vi "Find Table Boundaries.vi"(8 "error in (no error)":errorcluster, 11 "Configuration in":refnum<class "Configuration.lvclass">) -> (0 "error out":errorcluster, 3 "Configuration out":refnum<class "Configuration.lvclass">)   [LabVIEW 2023, in "Configuration.lvlib" / "Configuration.lvclass"]
doc: "Search the raw signal list data for the device handle, read the row and column definition fields, this defines the boundary of the device defintion table."
uses:
  Library/Configuration.lvclass
  Library/Configuration.lvclass/Configuration.ctl
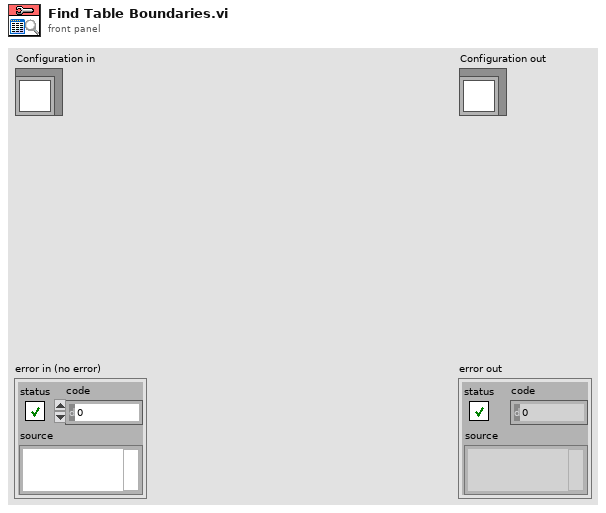
[diagram p1: front panel]
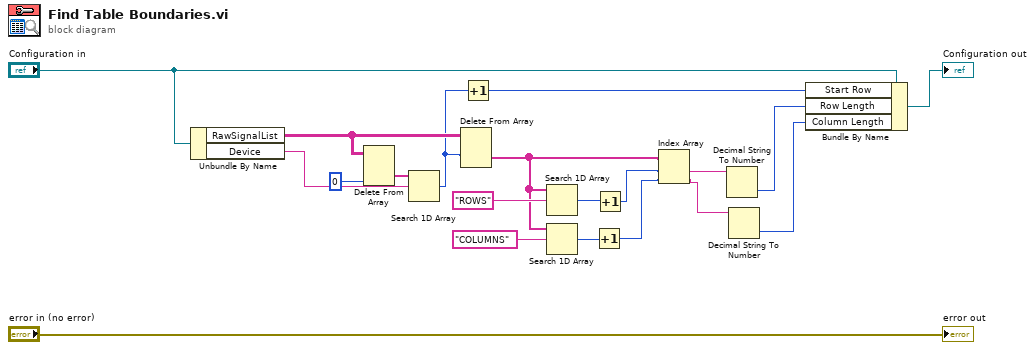
[diagram p0: block diagram]
diagram:
  n1 = Unbundle By Name("Configuration in") -> ("RawSignalList"=w17:string[][], "Device"=w1:string)
  n2 = Delete From Array(array=w17, index (col)=0 ("disabled index (col)")) -> (deleted portion=w18:string[])  [unwired: 2 in, 1 out]
  n3 = Search 1D Array(1D array=w18, element=w1) -> (index of element=w8:i32)  [unwired: 1 in]
  n4 = Delete From Array(array=w17, index (row)=w8) -> (deleted portion=w12:string[])  [unwired: 2 in, 1 out]
  n5 = Increment(x=w8) -> (x+1=w7:i32)
  n6 = Search 1D Array(1D array=w12, element="ROWS") -> (index of element=w14:i32)  [unwired: 1 in]
  n7 = Search 1D Array(1D array=w12, element="COLUMNS") -> (index of element=w13:i32)  [unwired: 1 in]
  n8 = Increment(x=w13) -> (x+1=w5:i32)
  n9 = Increment(x=w14) -> (x+1=w6:i32)
  n10 = Index Array(array=w12, index #1=w6, index #2=w5) -> (element #1=w11:string, element #2=w10:string)
  n11 = Decimal String To Number(string=w11) -> (number=w4:i32)  [unwired: 2 in, 1 out]
  n12 = Decimal String To Number(string=w10) -> (number=w3:i32)  [unwired: 2 in, 1 out]
  n13 = Bundle By Name(cluster="Configuration in", "Start Row"=w7, "Row Length"=w4, "Column Length"=w3) -> (→"Configuration out":refnum<class "Configuration.lvclass">)
  "error out" <- "error in (no error)"
